vi "BrightnessShift.vi"(9 "Cluster in":cluster{i32, i32, i32}, 10 "Image Pixels (U32)":u32[][](array[numeric]), 11 "Image Pixels (U32) 2":u32[][](array[numeric])) -> (3 "Cluster out":cluster{i32, i32, i32})   [LabVIEW 2019]
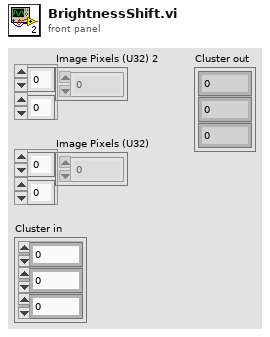
[diagram p1: front panel]
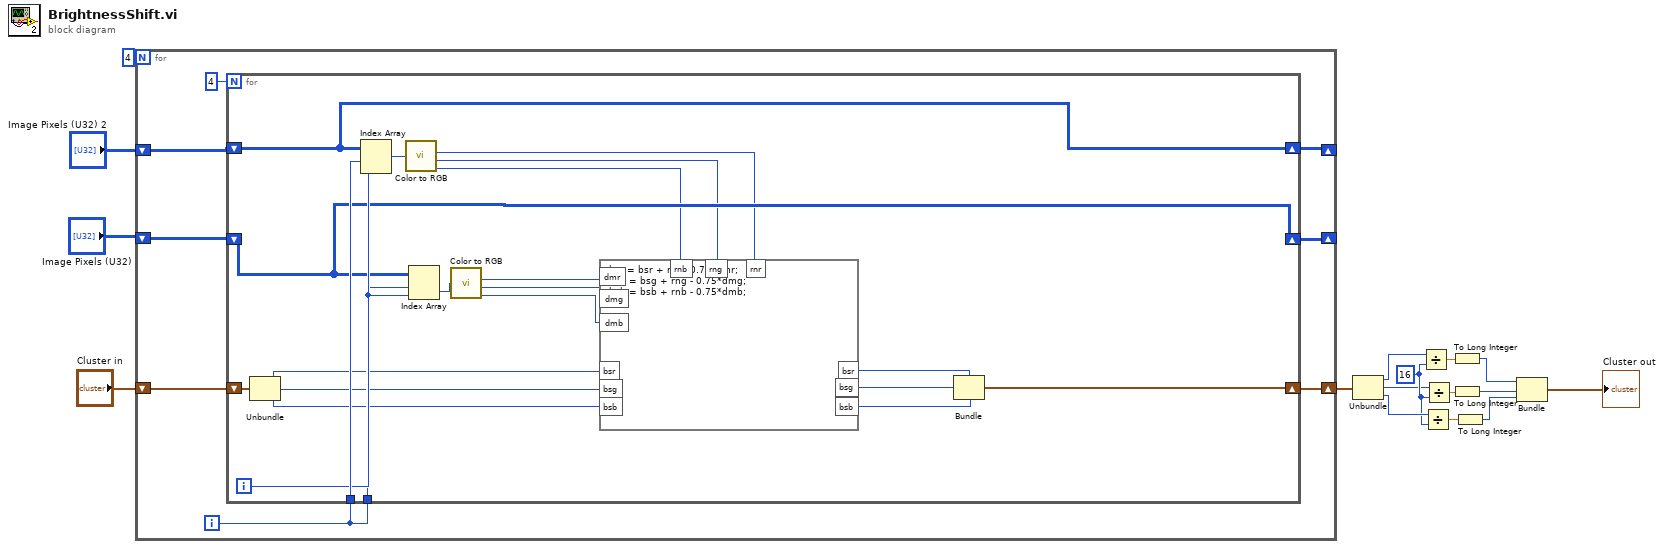
[diagram p0: block diagram]
diagram:
  w8 = 16 ("y")
  n1 = for {
    N: 4 -> [_]
    shift-right: [w23] -> _
    shift-left: "Image Pixels (U32) 2" -> [w24]
    shift-right: [w20] -> _
    shift-left: "Image Pixels (U32)" -> [w22]
    shift-right: [w17] -> w5
    shift-left: "Cluster in" -> [w18]
    i -> [w21]
    n2 = for {
      N: 4 -> [_]
      shift-right: [w42] -> w23
      shift-left: w24 -> [w42]
      tunnel: w21 -> [w45]
      shift-right: [w41] -> w20
      shift-left: w22 -> [w41]
      tunnel: w21 -> [w43]
      shift-right: [w25] -> w17
      shift-left: w18 -> [w39]
      i -> [w44]
      n3 = Unbundle(w39) -> (w38:i32, w37:i32, w36:i32)
      n4 = Index Array(array=w42, index (row)=w45, index (col)=w44) -> (element=w40:u32)
      n5 = call <vilib>:"Color to RGB.vi"("Color"=w40) -> ("R"=w31:u8, "G"=w30:u8, "B"=w29:u8)  [unwired: 1 out]
      n6 = Index Array(array=w41, index (row)=w43, index (col)=w44) -> (element=w35:u32)
      n7 = call <vilib>:"Color to RGB.vi"("Color"=w35) -> ("R"=w34:u8, "G"=w33:u8, "B"=w32:u8)  [unwired: 1 out]
      n8 = formula code="bsr = bsr + rnr - 0.75*dmr;\nbsg = bsg + rng - 0.75*dmg;\nbsb = bsb + rnb - 0.75*dmb;"("bsr"=w38, "bsg"=w37, "bsb"=w36, "rnb"=w29, "rng"=w30, "rnr"=w31, "dmr"=w34, "dmg"=w33, "dmb"=w32) -> ("bsr"=w28:i32, "bsg"=w27:i32, "bsb"=w26:i32)
      n9 = Bundle("bsr"=w28, "bsg"=w27, "bsb"=w26) -> (w25:cluster{"bsr":i32, "bsg":i32, "bsb":i32})  [unwired: 1 in]
    }
  }
  n10 = Unbundle(w5) -> (w6:i32, w7:i32, w9:i32)
  n11 = Divide(x=w6, y=w8) -> (x/y=w12:dbl)
  n12 = Divide(x=w9, y=w8) -> (x/y=w10:dbl)
  n13 = Divide(x=w7, y=w8) -> (x/y=w11:dbl)
  n14 = To Long Integer(number=w12) -> (32bit integer=w13:i32)
  n15 = To Long Integer(number=w11) -> (32bit integer=w14:i32)
  n16 = To Long Integer(number=w10) -> (32bit integer=w15:i32)
  n17 = Bundle(w13, w14, w15) -> (→"Cluster out":cluster{i32, i32, i32})  [unwired: 1 in]
